vi "Malleable to Polymorphic.vi"(8 "error in (no error)":errorcluster, 10 "Polymorphic Templates Path":path, 11 "Library Ref In":refnum<vi>) -> (0 "error out":errorcluster, 3 "Library Ref Out":refnum<vi>)   [LabVIEW 2020]
doc: "Replaces all malleable VIs in this library with polymorphic instances generated from VIs in Polymorphic Templates Path."
uses:
  <vilib>/Utility/traverseref.llb/TRef TravTarget.ctl
  b1d83953-403a-4f8f-8a0b-46b8d1093b65.vi
  Global.vi
  <vilib>/Utility/traverseref.llb/VI Scripting - Traverse.lvlib
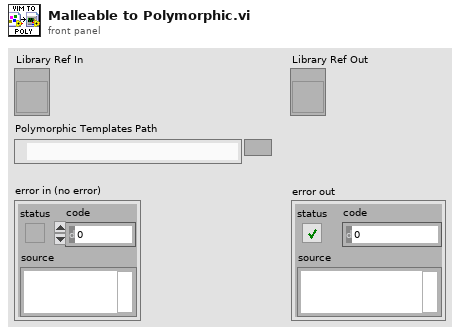
[diagram p1: front panel]
types:
  T1 = typedef "TRef TravTarget.ctl" = enum16{"FP", "BD", "Other"}
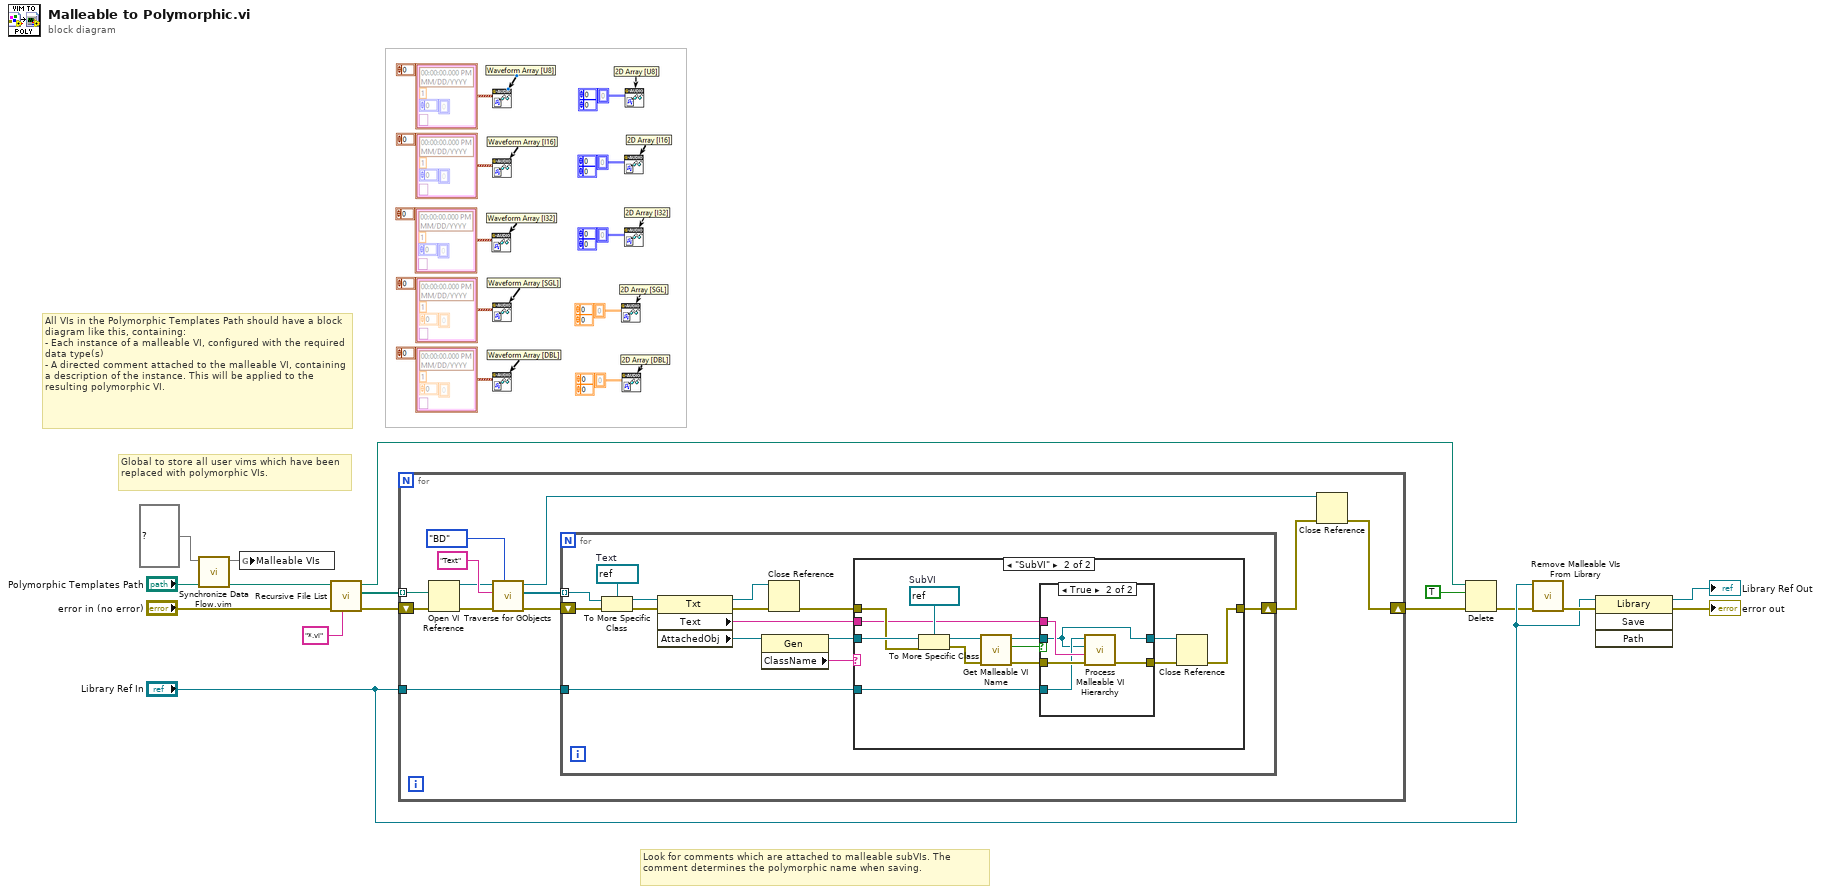
[diagram p0: block diagram]
diagram:
  # "All VIs in the Polymorphic Templates Path should have a block diagram like this, containing:\n- Each instance of a malleable VI, configured with the required data type(s)\n- A directed comment attached to the malleable VI, containing a description of the instance. This will be applied to the resulting polymorphic VI."
  # "Look for comments which are attached to malleable subVIs. The comment determines the polymorphic name when saving."
  # "Global to store all user vims which have been replaced with polymorphic VIs."
  n1 = call "Synchronize Data Flow.vim"("input 4"="Polymorphic Templates Path", "input 1"=set{string} {} ("Malleable VIs")) -> ("output 4"=w8:path, "output 1"=w10:set{string})  [unwired: 2 in, 2 out]
  n2 = global write "Global.vi" "Malleable VIs"(w10) -> ()
  n3 = call <vilib>:"Recursive File List.vi"("pattern"="*.vi", "error in (no error)"="error in (no error)", "Folder Path"=w8) -> ("error out"=w14:errorcluster, "All Files in Dir"=w15:path[], "dup Folder Path"=w6:path)  [unwired: 4 in, 2 out]
  n4 = for {
    tunnel: w15 -> [w28] mode=indexing
    shift-right: [w25] -> w4
    shift-left: w14 -> [w27]
    tunnel: "Library Ref In" -> [w26]
    n5 = Open VI Reference(vi path=w28, error in (no error)=w27) -> (vi reference=w22:refnum<vi>, error out=w19:errorcluster)  [unwired: 4 in]
    n6 = call <vilib>:"Traverse for GObjects.vi"("Traverse Target"=TRef_TravTarget."BD", "error in (no error)"=w19, "Class Name"="Text", "VI Refnum"=w22) -> ("error out"=w18:errorcluster, "References"=w20:refnum<vi>[], "dup VI Refnum"=w21:refnum<vi>)  [unwired: 4 in, 1 out]
    n7 = for {
      tunnel: w20 -> [w30] mode=indexing
      shift-right: [w42] -> w17
      shift-left: w18 -> [w29]
      tunnel: w26 -> [w41]
      w40 = refnum<vi> refnum  # Text
      n8 = To More Specific Class(target class=w40, reference=w30, error in=w29) -> (specific class reference=w39:refnum<vi>, error out=w35:errorcluster)
      n9 = property class="Txt"(reference=w39, error in=w35) -> (reference out=w33:refnum<vi>, error out=w32:errorcluster, "Text"=w34:string, "AttachedObj"=w38:refnum<vi>)
      n10 = property class="Gen"(reference=w38) -> (reference out=w36:refnum<vi>, "ClassName"=w37:string)  [unwired: 1 in, 1 out]
      n11 = Close Reference(reference=w33, error in (no error)=w32) -> (error out=w31:errorcluster)
      n12 = case shown="\"SubVI\"" w37 {
        tunnel: w36 -> [_ w56]
        tunnel: w34 -> [_ w49]
        tunnel: [w43 w45] -> w42
        tunnel: w31 -> [w43 w50]
        tunnel: w41 -> [_ w48]
        frame Default {
          # "Label not attached to subVI, ignore."
        }
        frame "SubVI" {
          w55 = refnum<vi> refnum  # SubVI
          n13 = To More Specific Class(target class=w55, reference=w56, error in=w50) -> (specific class reference=w53:refnum<vi>, error out=w52:errorcluster)
          n14 = call "Get Malleable VI Name.vi"("error in (no error)"=w52, "SubVI Ref In"=w53) -> ("error out"=w51:errorcluster, "Is Malleable VI?"=w47:bool, "SubVI Ref Out"=w54:refnum<vi>)  [unwired: 5 in, 2 out]
          n15 = case shown="True" w47 {
            tunnel: w54 -> [w57 w59]
            tunnel: w51 -> [w58 w63]
            tunnel: [w58 w62] -> w46
            tunnel: w49 -> [_ w61]
            tunnel: w48 -> [_ w60]
            tunnel: [w57 w59] -> w44
            frame False {
            }
            frame True {
              n16 = call "Process Malleable VI Hierarchy.vi"("error in (no error)"=w63, "Polymorphic Label"=w61, "SubVI Ref In"=w59, "Library Ref In"=w60) -> ("error out"=w62:errorcluster)  [unwired: 7 in]
            }
          }
          n17 = Close Reference(reference=w44, error in (no error)=w46) -> (error out=w45:errorcluster)
        }
      }
    }
    n18 = Close Reference(reference=w21, error in (no error)=w17) -> (error out=w25:errorcluster)
  }
  n19 = Delete(path (use dialog)=w6, entire hierarchy (F)=TRUE, error in=w4) -> (error out=w3:errorcluster)  [unwired: 2 in, 2 out]
  n20 = call "Remove Malleable VIs From Library.vi"("error in (no error)"=w3, "Library Ref"="Library Ref In") -> ("error out"=w12:errorcluster)  [unwired: 9 in]
  n21 = invoke class="Library" method="Save"(reference="Library Ref In", error in=w12) -> (reference out=→"Library Ref Out":refnum<vi>, error out=→"error out":errorcluster)  [unwired: 2 in, 2 out]
